vi "findFromList.vi"(8 "error in (no error)":errorcluster, 10 "Path":path, 11 "CompiledList in":refnum<class "CompiledList.lvclass">) -> (0 "error out":errorcluster, 1 "found?":bool, 2 "CompiledScript":T1, 3 "CompiledList out":refnum<class "CompiledList.lvclass">)   [LabVIEW 2011, in "Compiler.lvlib" / "CompiledList.lvclass"]
uses:
  CompiledList.lvclass
  ScriptListCompiler/ScriptListCompiler.lvclass
  Hal/Channels/VoltOutput/AnalogOutput.lvclass
  Hal/Channels/Digital/DigitalOutput.lvclass
  Hal/Channels/DDSOutput/Generic/DDSOutput.lvclass
  CompiledList.lvclass/CompiledList.ctl
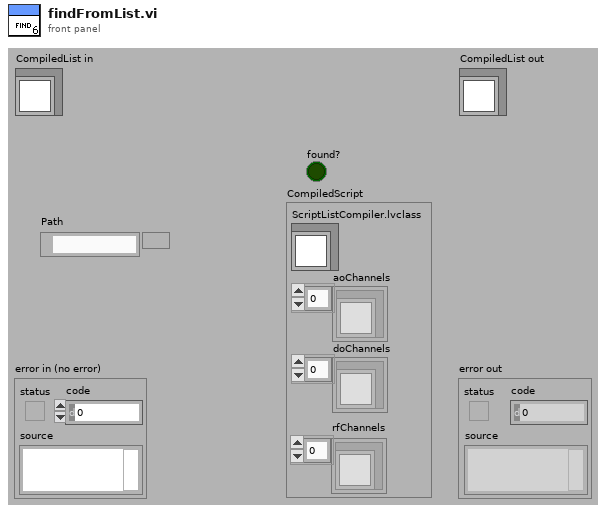
[diagram p1: front panel]
types:
  T1 = cluster{"ScriptListCompiler.lvclass":refnum<class "ScriptListCompiler.lvclass">, "aoChannels":refnum<class "AnalogOutput.lvclass">[], "doChannels":refnum<class "DigitalOutput.lvclass">[], "rfChannels":refnum<class "DDSOutput.lvclass">[]}
  T2 = cluster{"ScriptListCompiler.lvclass":refnum<class "ScriptListCompiler.lvclass">, "aoChannels":refnum<class "AnalogOutput.lvclass">[], "doChannels":refnum<class "DigitalOutput.lvclass">[], "rfChannels":refnum<class "DDSOutput.lvclass">[]}[]
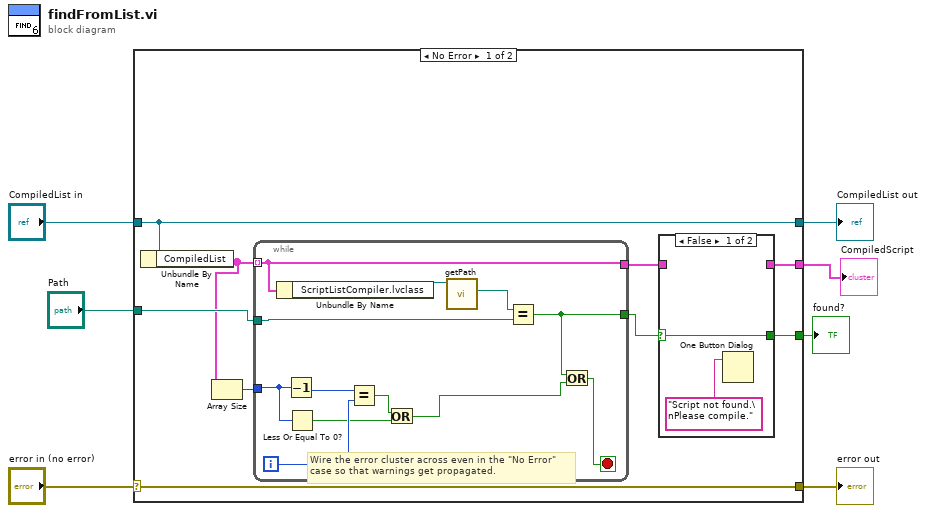
[diagram p0: block diagram]
diagram:
  n1 = case shown="No Error" "error in (no error)" {
    selector: "error in (no error)" -> [w16 w34]
    tunnel: [w16 w34] -> w6
    tunnel: [w15 w33] -> w4
    tunnel: "CompiledList in" -> [w15 w33]
    tunnel: "Path" -> [w14 _]
    tunnel: [w9 _] -> w1
    tunnel: [w8 _] -> w2
    frame No Error {
      # "Wire the error cluster across even in the \"No Error\"\ncase so that warnings get propagated."
      n2 = Unbundle By Name(w15) -> ("CompiledList"=w13:T2)
      n3 = Array Size(array=w13) -> (size(s)=w12:i32)
      n4 = while {
        tunnel: w13 -> [w25] mode=indexing
        tunnel: w14 -> [w30]
        tunnel: w12 -> [w24]
        tunnel: [w26] -> w11
        tunnel: [w25] -> w10
        i -> [w28]
        stop <- w27 stop-if-true
        n5 = Unbundle By Name(w25) -> ("ScriptListCompiler.lvclass"=w32:refnum<class "ScriptListCompiler.lvclass">)
        n6 = Decrement(x=w24) -> (x-1=w29:i32)
        n7 = Less Or Equal To 0?(x=w24) -> (x <= 0?=w23:bool)
        n8 = Equal?(x=w29, y=w28) -> (x = y?=w22:bool)
        n9 = Or(x=w22, y=w23) -> (x .or. y?=w21:bool)
        n10 = call "getPath.vi"("ScriptListCompiler in"=w32) -> ("Path"=w31:path)  [unwired: 8 in, 2 out]
        n11 = Equal?(x=w31, y=w30) -> (x = y?=w26:bool)
        n12 = Or(x=w26, y=w21) -> (x .or. y?=w27:bool)
      }
      n13 = case shown="False" w11 {
        selector: w11 -> [w17 w19]
        tunnel: w10 -> [_ w20]
        tunnel: [_ w20] -> w9
        tunnel: [w17 w19] -> w8
        frame False {
          n14 = One Button Dialog(message="Script not found.\nPlease compile.") -> ()  [unwired: 1 in, 1 out]
        }
        frame True {
        }
      }
    }
    frame Error {
    }
  }
  "error out" <- w6
  "CompiledList out" <- w4
  "found?" <- w2
  "CompiledScript" <- w1
